vi "AccuracyResultQuery.vi"(8 "error in (no error)":errorcluster, 10 "pulMHMHandle":u32, 11 "pulNumberOfBytes":u32) -> (0 "error out":errorcluster, 1 "XY Graph":cluster{dbl[], dbl[]}[](graph) caption="Calibration Curves", 2 "Error Range":dbl caption="degree" format="%.03f%.;", 3 "Error_bit":dbl caption="bit" format="%.03f%.;", 5 "Revolutions":dbl step=1.0)   [LabVIEW 2017]
uses:
  DUT_Interface/lv_interface/enums/MHM_CalDataEnum.ctl
  DUT_Interface/lv_interface/MHM_1SL_interface.lvlib
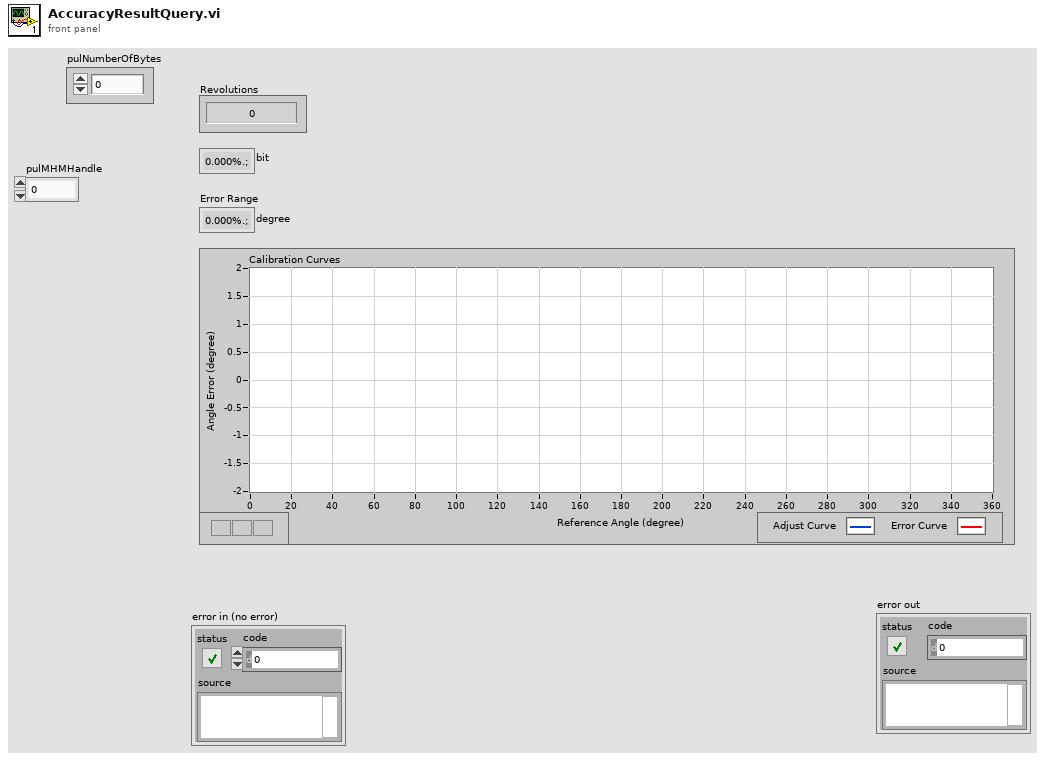
[diagram p1: front panel]
types:
  T1 = typedef "MHM_CalDataEnum.ctl" = enum16{"MHM_DUTRAW", "MHM_DUTCONT", "MHM_REFCONT", "MHM_DUTERR", "MHM_ADJERR", "MHM_REFRAW"}
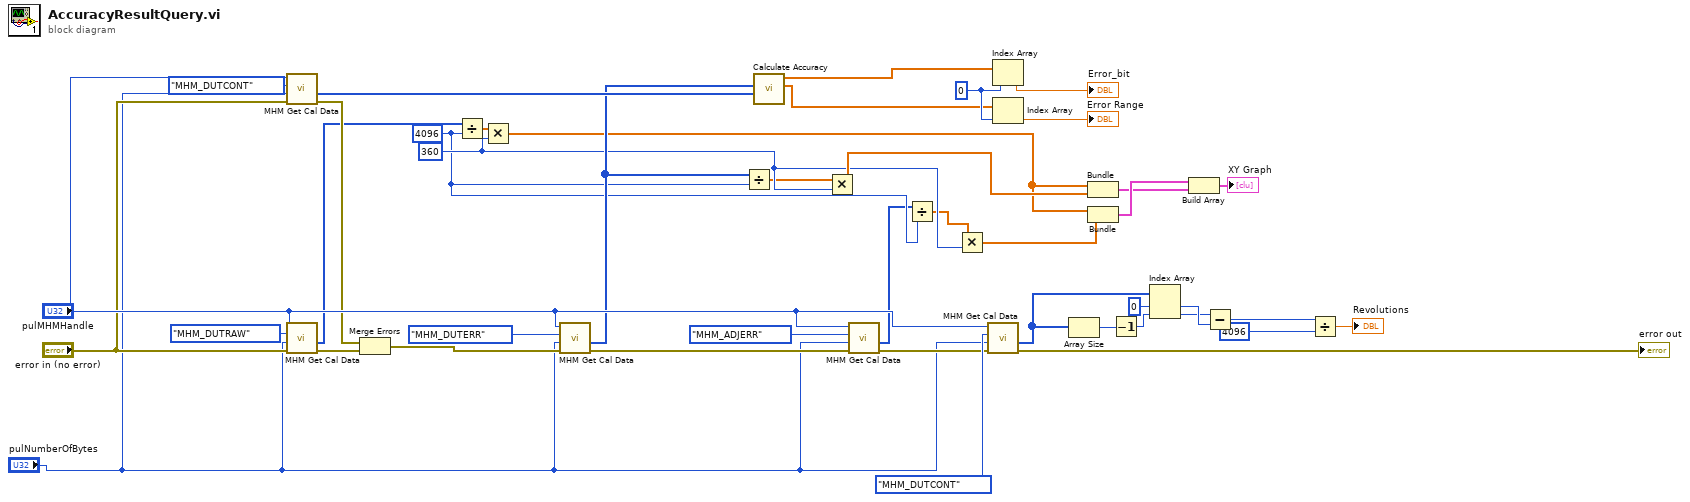
[diagram p0: block diagram]
diagram:
  w24 = 0 ("index")
  w12 = 360
  w11 = 4096
  n1 = call "MHM Get Cal Data.vi"("error in (no error)"="error in (no error)", "pulNumberOfBytes"="pulNumberOfBytes", "ulParam"=MHM_CalDataEnum."MHM_DUTCONT" ("MHM_CalDataEnum"), "ulMHMHandle"="pulMHMHandle") -> ("error out"=w28:errorcluster, "plData"=w27:i32[])  [unwired: 4 in, 2 out]
  n2 = call "MHM Get Cal Data.vi"("error in (no error)"="error in (no error)", "pulNumberOfBytes"="pulNumberOfBytes", "ulParam"=MHM_CalDataEnum."MHM_DUTRAW" ("MHM_CalDataEnum"), "ulMHMHandle"="pulMHMHandle") -> ("error out"=w29:errorcluster, "plData"=w19:i32[])  [unwired: 4 in, 2 out]
  n3 = Merge Errors(w28, w29) -> (w30:errorcluster)
  n4 = Divide(x=w19, y=w11) -> (x/y=w6:dbl[])
  n5 = Multiply(x=w6, y=w12) -> (x*y=w8:dbl[])
  n6 = call "MHM Get Cal Data.vi"("error in (no error)"=w30, "pulNumberOfBytes"="pulNumberOfBytes", "ulParam"=MHM_CalDataEnum."MHM_DUTERR" ("MHM_CalDataEnum"), "ulMHMHandle"="pulMHMHandle") -> ("error out"=w2:errorcluster, "plData"=w18:i32[])  [unwired: 4 in, 2 out]
  n7 = Divide(x=w18, y=w11) -> (x/y=w7:dbl[])
  n8 = call "Calculate Accuracy.vi"("CAL_DUT_CONT"=w27, "CAL_DUT_ERR"=w18) -> ("Accuracy [Degree]"=w22:dbl[], "Accuracy [Bit]"=w20:dbl[])  [unwired: 6 in, 2 out]
  n9 = Multiply(x=w7, y=w12) -> (x*y=w15:dbl[])
  n10 = call "MHM Get Cal Data.vi"("error in (no error)"=w2, "pulNumberOfBytes"="pulNumberOfBytes", "ulParam"=MHM_CalDataEnum."MHM_ADJERR" ("MHM_CalDataEnum"), "ulMHMHandle"="pulMHMHandle") -> ("error out"=w31:errorcluster, "plData"=w10:i32[])  [unwired: 4 in, 2 out]
  n11 = Divide(x=w10, y=w11) -> (x/y=w9:dbl[])
  n12 = Multiply(x=w9, y=w12) -> (x*y=w13:dbl[])
  n13 = call "MHM Get Cal Data.vi"("error in (no error)"=w31, "pulNumberOfBytes"="pulNumberOfBytes", "ulParam"=MHM_CalDataEnum."MHM_DUTCONT" ("MHM_CalDataEnum"), "ulMHMHandle"="pulMHMHandle") -> ("error out"=→"error out":errorcluster, "plData"=w34:i32[])  [unwired: 4 in, 2 out]
  n14 = Index Array(array=w20, index=w24) -> (element=→"Error_bit":dbl)
  n15 = Index Array(array=w22, index=w24) -> (element=→"Error Range":dbl)
  n16 = Array Size(array=w34) -> (size(s)=w36:i32)
  n17 = Bundle(w8, w15) -> (w16:cluster{dbl[], dbl[]})  [unwired: 1 in]
  n18 = Bundle(w8, w13) -> (w17:cluster{dbl[], dbl[]})  [unwired: 1 in]
  n19 = Decrement(x=w36) -> (x-1=w37:i32)
  n20 = Index Array(array=w34, index #1=0 ("index"), index #2=w37) -> (element #1=w39:i32, element #2=w38:i32)
  n21 = Build Array(w17, w16) -> (→"XY Graph":cluster{dbl[], dbl[]}[])
  n22 = Subtract(x=w38, y=w39) -> (x-y=w41:i32)
  n23 = Divide(x=w41, y=4096) -> (x/y=→"Revolutions":dbl)
